vi "test2.vi"() -> ()   [LabVIEW 2019]
panel:
  in  "write buffer":string
  in  "VISA resource name":refnum<visa-resource-name>
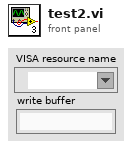
[diagram p1: front panel]
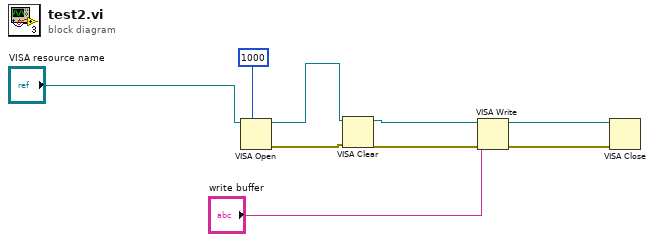
[diagram p0: block diagram]
diagram:
  n1 = VISA Open(timeout (0)=u32 1000 ("VISA Open timeout (0)"), VISA resource name="VISA resource name") -> (VISA resource name=w2:refnum<visa-resource-name>, error out=w4:errorcluster)  [unwired: 3 in]
  n2 = VISA Clear(VISA resource name=w2, error in (no error)=w4) -> (VISA resource name out=w1:refnum<visa-resource-name>, error out=w3:errorcluster)
  n3 = VISA Write(VISA resource name=w1, write buffer="write buffer", error in (no error)=w3) -> (VISA resource name out=w7:refnum<visa-resource-name>, error out=w6:errorcluster)  [unwired: 1 out]
  n4 = VISA Close(VISA resource name=w7, error in (no error)=w6) -> ()  [unwired: 1 out]
